vi "Main.vi"() -> ()   [LabVIEW 2013]
uses:
  <vilib>/myRIO/Common/Instrument Driver Framework/myRIO v1.0/UART/vis/myRIO v1.0 Close UART.vi
  <vilib>/myRIO/Common/Instrument Driver Framework/Utilities/vis/FPGA Ref Manager.vi
  <vilib>/myRIO/Common/Instrument Driver Framework/myRIO v1.0/myRIO v1.0 Reset FPGA.vi
  <vilib>/myRIO/Instrument Drivers/Utilities/Utilities.lvlib
panel:
  out "LCD display":string
  in  "[ESC]":bool
  # "LCD (UART) demo"
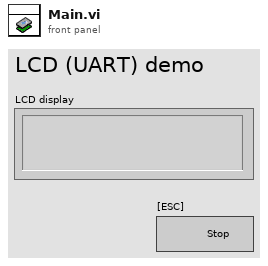
[diagram p1: front panel]
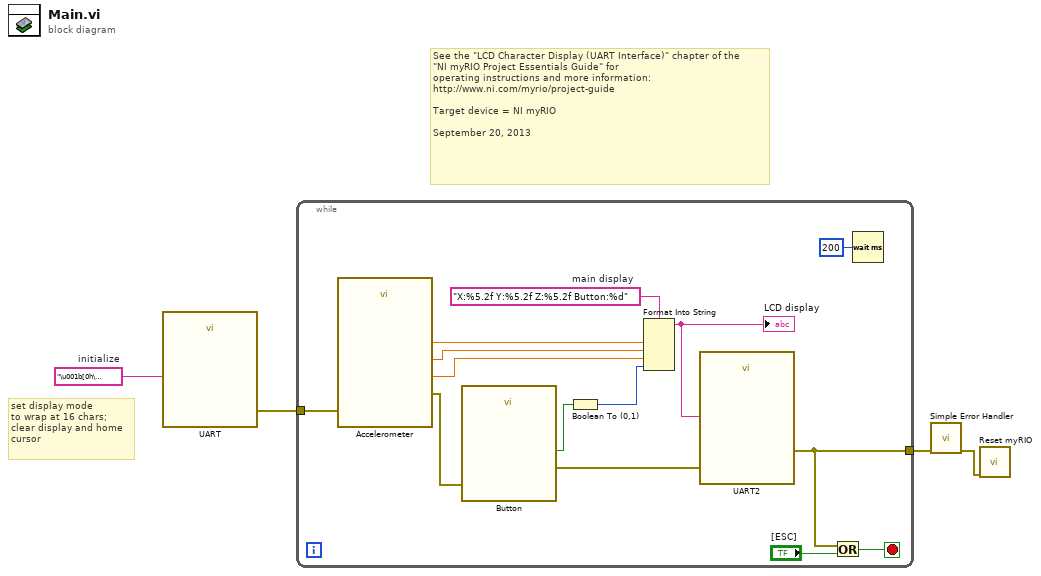
[diagram p0: block diagram]
diagram:
  w1 = "\u001b[0h\u001b[j"  # initialize
  # "See the \"LCD Character Display (UART Interface)\" chapter of the\n\"NI myRIO Project Essentials Guide\" for\noperating instructions and more information: \nhttp://www.ni.com/myrio/project-guide\n\nTarget device = NI myRIO\n\nSeptember 20, 2013"
  # "set display mode\nto wrap at 16 chars;\nclear display and home\ncursor"
  n1 = call "UART"("Characters to Write"=w1) -> ("error out"=w4:errorcluster)  [unwired: 25 in, 1 out]
  n2 = while {
    tunnel: w4 -> [w16]
    tunnel: [w6] -> w2
    stop <- w8 stop-if-true
    w18 = "X:%5.2f Y:%5.2f Z:%5.2f Button:%d"  # main display
    n3 = call "Accelerometer"("error in (no error)"=w16) -> ("X-Axis"=w15:dbl, "Y-Axis"=w14:dbl, "Z-Axis"=w13:dbl, "error out"=w12:errorcluster)  [unwired: 23 in]
    n4 = call "Button"("error in (no error)"=w12) -> ("Value"=w11:bool, "error out"=w9:errorcluster)  [unwired: 25 in]
    n5 = Boolean To (0,1)(Boolean=w11) -> (0, 1=w17:i16)
    n6 = Format Into String "Format Into String"(format string=w18, w15, w14, w13, w17) -> (resulting string=w5:string)  [unwired: 2 in, 1 out]
    "LCD display" <- w5
    n7 = call "UART2"("Characters to Write"=w5, "error in (no error)"=w9) -> ("error out"=w6:errorcluster)  [unwired: 24 in, 1 out]
    n8 = Or(x=w6, y="[ESC]") -> (x .or. y?=w8:bool)
    n9 = Wait (ms)(milliseconds to wait=u32 200) -> ()  [unwired: 1 out]
  }
  n10 = call <vilib>:"Simple Error Handler.vi"("error in (no error)"=w2) -> ("error out"=w3:errorcluster)  [unwired: 4 in, 4 out]
  n11 = call <vilib>:"Reset myRIO.vi"("error in (no error)"=w3) -> ()  [unwired: 10 in, 1 out]
